vi "Get Size.vi"(8 "error in (no error)":errorcluster, 11 "Glyph Destination in":refnum<class "Listbox Icon Canvas.lvclass">) -> (0 "error out":errorcluster, 2 "Size":cluster{"Width":u16, "Height":u16}, 3 "Glyph Destination out":refnum<class "Listbox Icon Canvas.lvclass">)   [LabVIEW 2023, in "Font Glyph Drawer Interface.lvlib" / "Listbox Icon Canvas.lvclass"]
uses:
  Listbox Icon Canvas.lvclass
  Listbox Icon Canvas.lvclass/Listbox Icon Canvas.ctl
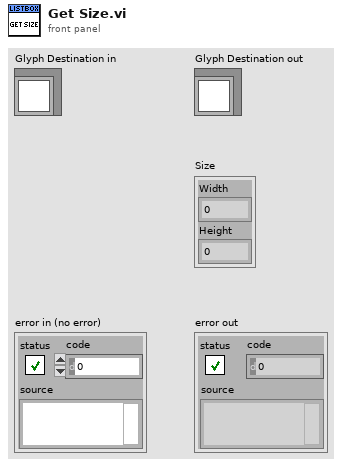
[diagram p1: front panel]
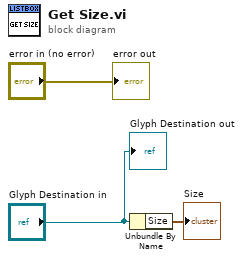
[diagram p0: block diagram]
diagram:
  n1 = Unbundle By Name("Glyph Destination in") -> ("Size"=→"Size":cluster{"Width":u16, "Height":u16})
  "error out" <- "error in (no error)"
  "Glyph Destination out" <- "Glyph Destination in"
